vi "Setup.vi"(8 "error in (no error)":errorcluster, 11 "Configuration File Interface Test In":refnum<class "Configuration File Base Interface Test.lvclass">) -> (0 "error out":errorcluster, 3 "Configuration File Interface Test Out":refnum<class "Configuration File Base Interface Test.lvclass">)   [LabVIEW 2020, in "Configuration File Base Interface Test.lvclass"]
uses:
  Configuration File Base Interface Test.lvclass
  Configuration Interface Test/Configuration Interface Test.lvclass
  Mock Configurable Base/Mock Configurable Base.lvclass
  C:/Git/triarc-framework/source/Framework/Base/Base.lvclass
  C:/Git/triarc-framework/source/Framework/Configuration File/Configuration File.lvclass
  C:/Git/triarc-framework/source/Framework/Configuration/Configuration.lvclass
  C:/Git/triarc-framework/source/Framework Test/Mock Configurable Base/Mock Configurable Base.lvclass
  C:/Git/triarc-framework/source/Framework Test/Configuration Interface Test/Configuration Interface Test.lvclass
  C:/Program Files (x86)/National Instruments/LabVIEW 2020/vi.lib/Astemes/LUnit/Test Case.lvclass
  C:/Git/triarc-framework/source/Framework Test/Configuration File Interface Test/Configuration File Base Interface Test.lvclass
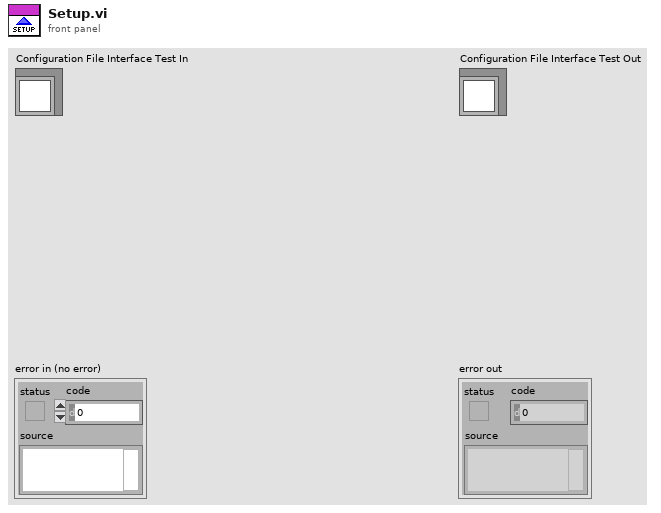
[diagram p1: front panel]
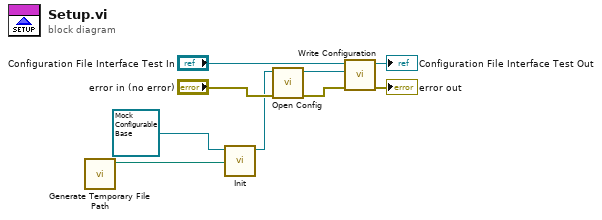
[diagram p0: block diagram]
diagram:
  n1 = call <vilib>:"Generate Temporary File Path.vi"() -> ("Unique Temporary File Path"=w1:path)  [unwired: 10 in, 1 out]
  n2 = call-dynamic "Init.vi"("Config File Path"=w1, "Base In"=refnum<class "Mock Configurable Base.lvclass"> refnum ("Mock Configurable.lvclass")) -> ("Base Out"=w2:refnum<class "Mock Configurable Base.lvclass">)  [unwired: 8 in, 1 out]
  n3 = call-dynamic "Open Config.vi"("error in (no error)"="error in (no error)", "Configuration File File In"=w2) -> ("error out"=w3:errorcluster, "Configuration File File Out"=w5:refnum<class "Mock Configurable Base.lvclass">)  [unwired: 7 in, 1 out]
  n4 = call "Write Configuration.vi"("error in (no error)"=w3, "Configuration"=w5, "Configuration Interface Test In"="Configuration File Interface Test In") -> ("error out"=→"error out":errorcluster, "Configuration Interface Test Out"=→"Configuration File Interface Test Out":refnum<class "Configuration File Base Interface Test.lvclass">)  [unwired: 7 in]
